vi "DIDOWhileLoop.vi"() -> ()   [LabVIEW 2020]
uses:
  <instrlib>/HandsOnPi2040/Public/DigOuts.ctl
  <instrlib>/HandsOnPi2040/Public/DigIns.ctl
  <instrlib>/HandsOnPi2040/HandsOnPi2040.lvlib
panel:
  out "Numeric":i32
  out "error out":errorcluster
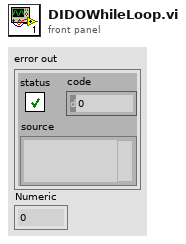
[diagram p1: front panel]
types:
  T1 = typedef "HandsOnPi2040.lvlib/DigIns.ctl" = enum16{"No DI - Error", "DI1 (GPIO7)", "DI2 (GPIO8)", "DI3 (GPIO9)", "DI4 (GPIO10)"}
  T2 = typedef "HandsOnPi2040.lvlib/DigOuts.ctl" = enum16{"No DO - Error", "DO1 (GPIO2)", "DO2 (GPIO3)", "DO3 (GPIO4)", "DO4 (GPIO5)", "BEEP (GPIO6)"}
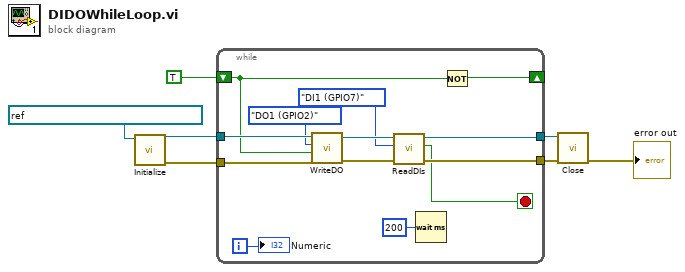
[diagram p0: block diagram]
diagram:
  n1 = call <instrlib>:"Initialize.vi"("VISA resource name"=refnum<visa-resource-name> "TCPIP0::10.0.2.15::6340::SOCKET") -> ("error out"=w7:errorcluster, "VISA resource name out"=w3:refnum<visa-resource-name>)  [unwired: 8 in, 1 out]
  n2 = while {
    tunnel: w7 -> [w20]
    tunnel: [w13] -> w6
    tunnel: [w14] -> w4
    tunnel: w3 -> [w19]
    shift-right: [w18] -> _
    shift-left: TRUE -> [w17]
    i -> [w11]
    stop <- w10 stop-if-true
    n3 = call <instrlib>:"WriteDO.vi"("error in (no error)"=w20, "DO Value (True)"=w17, "Output"=DigOuts."DO1 (GPIO2)", "VISA resource name"=w19) -> ("error out"=w16:errorcluster, "VISA resource name out"=w15:refnum<visa-resource-name>)  [unwired: 6 in]
    n4 = call <instrlib>:"ReadDIs.vi"("error in (no error)"=w16, "Digital Inputs"=DigIns."DI1 (GPIO7)", "VISA resource name"=w15) -> ("error out"=w13:errorcluster, "DIStatus"=w10:bool, "VISA resource name out"=w14:refnum<visa-resource-name>)  [unwired: 6 in]
    n5 = Wait (ms)(milliseconds to wait=u32 200) -> ()  [unwired: 1 out]
    n6 = Not(x=w17) -> (.not. x?=w18:bool)
    "Numeric" <- w11
  }
  n7 = call <instrlib>:"Close.vi"("error in (no error)"=w6, "VISA resource name"=w4) -> ("error out"=→"error out":errorcluster)  [unwired: 9 in]
